vi "Disable_Enable.vi"(7 "Disabled":T2(ring)=enum."Disabled and Grayed Out", 8 "error in (no error)":errorcluster, 10 "Command":T1=enum."INIT", 11 "EpiWrapper in":refnum<class "EpiWrapper.lvclass">) -> (0 "error out":errorcluster, 3 "EpiWrapper out":refnum<class "EpiWrapper.lvclass">)   [LabVIEW 2012, in "EpiWrapper.lvclass"]
uses:
  EpiWrapper.lvclass
  Controls/Command_Enum.ctl
  Controls/Control_Selector.ctl
  Controls/Input_Selector.ctl
  EpiWrapper.lvclass/EpiWrapper.ctl
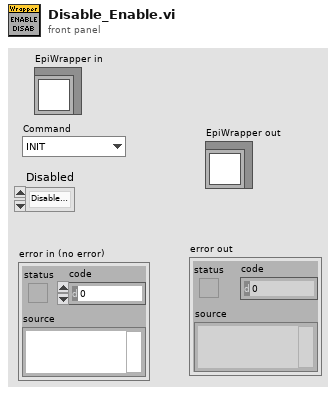
[diagram p1: front panel]
types:
  T1 = typedef "Command_Enum.ctl" = enum16{"RESETCONFIG", "OPENCONFIG", "RESET", "INIT", "LOAD", "MEASURE", "NEW", "SAVE", "UPDATE_INT", "SWAP_MODE", "UPDATE_ACQ", "EXIT", "CANCEL"}
  T2 = enum8{"Enabled", "Disabled", "Disabled and Grayed Out"}
  T3 = typedef "Input_Selector.ctl" = enum16{"Wafer ID", "Test", "New", "Save", "Load", "Cancel"}
  T4 = typedef "Control_Selector.ctl" = enum16{"Pass", "Fail", "Measure", "Area", "TestData"}
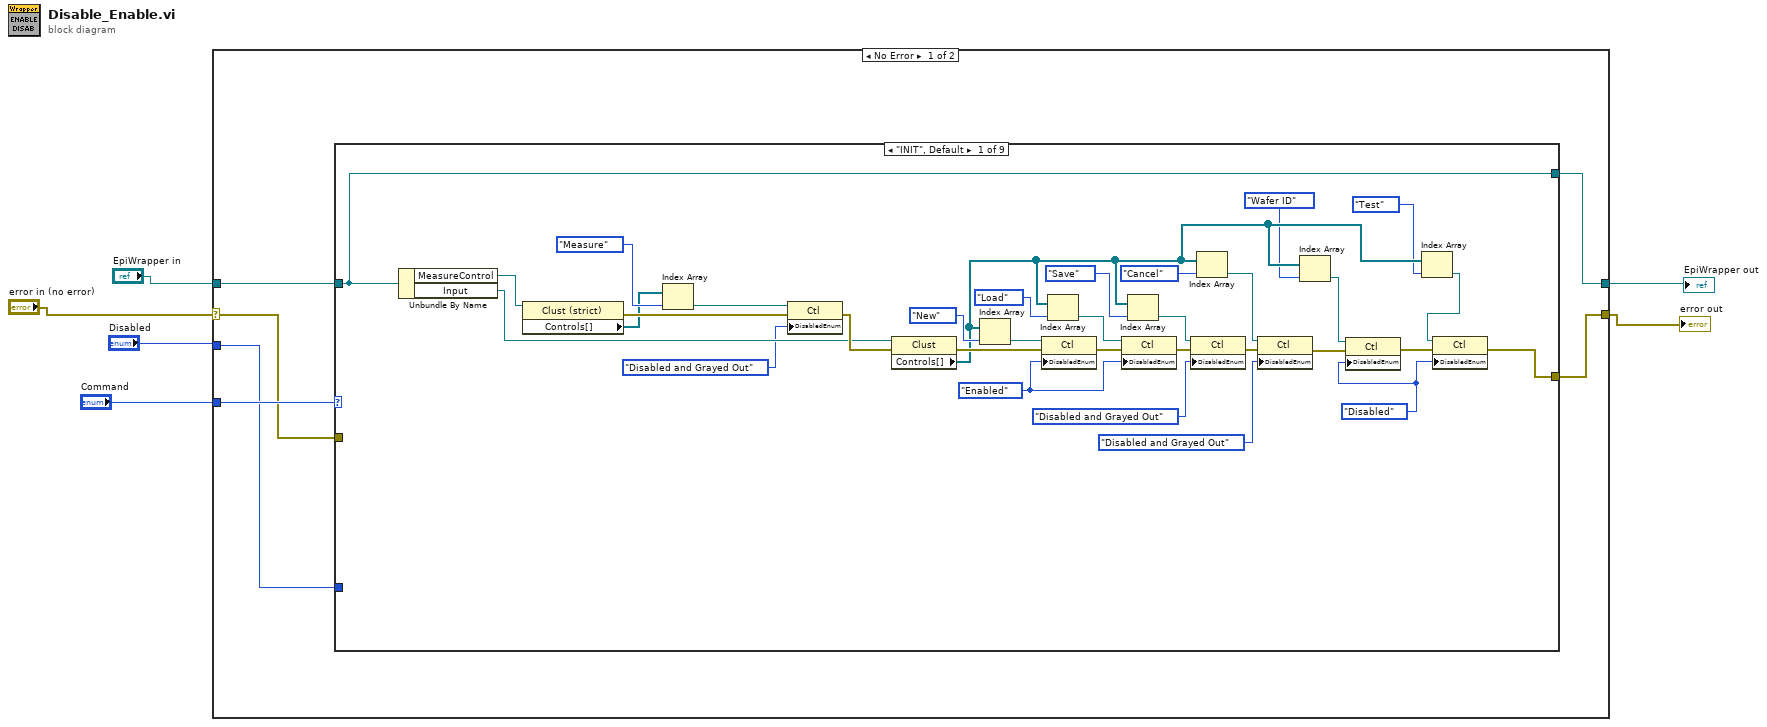
[diagram p0: block diagram]
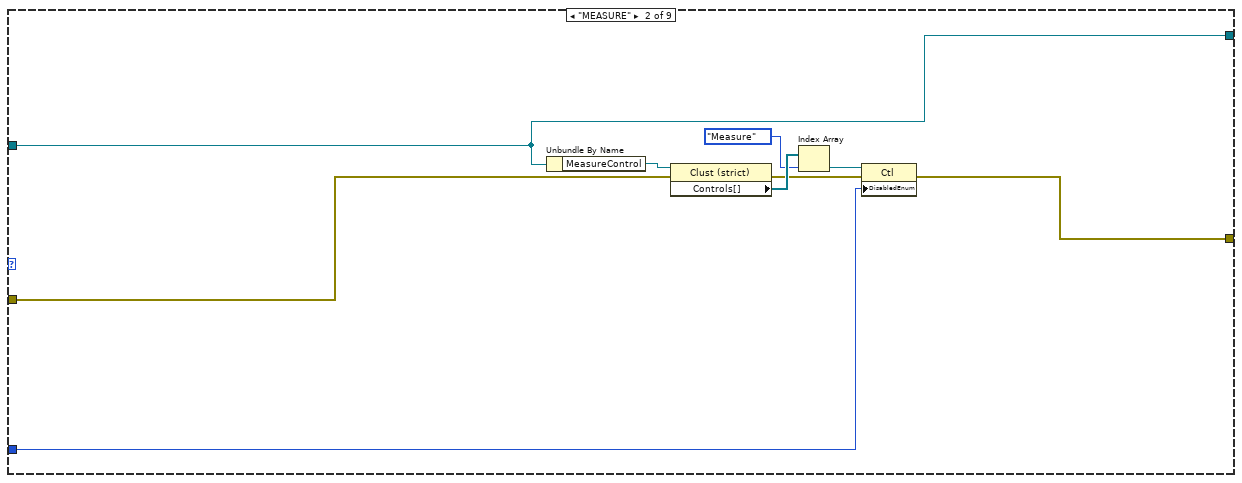
[diagram p2: hidden frame]
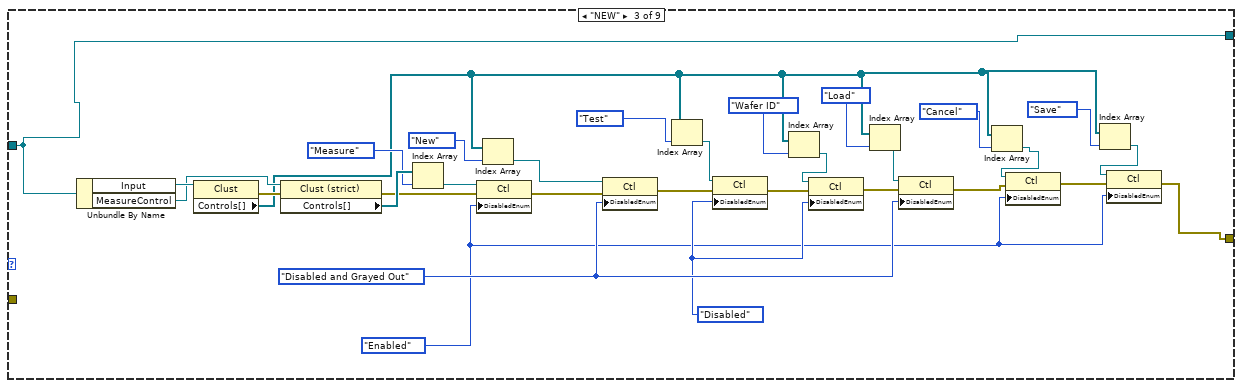
[diagram p3: hidden frame]
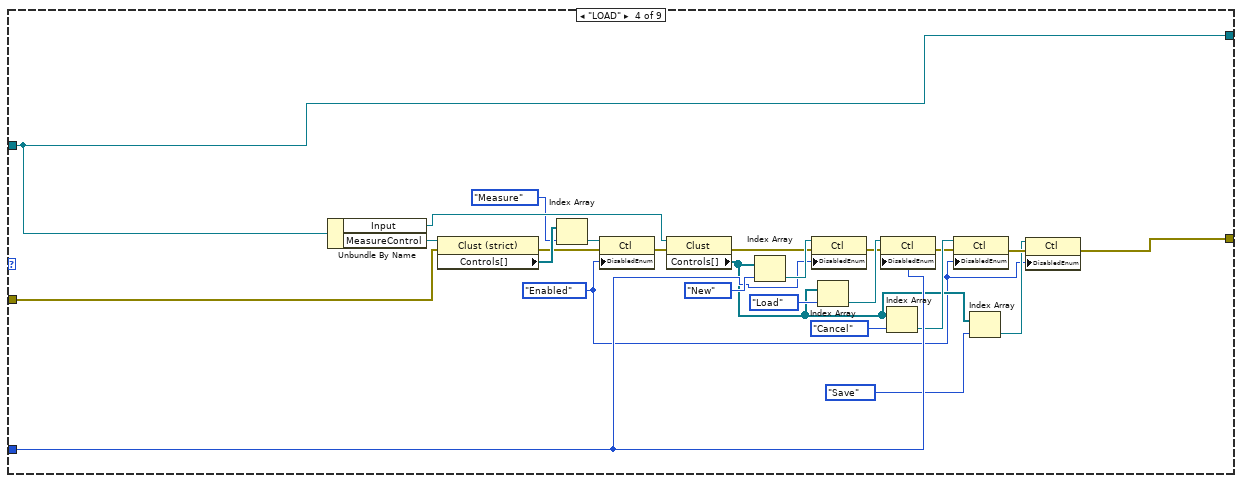
[diagram p4: hidden frame]
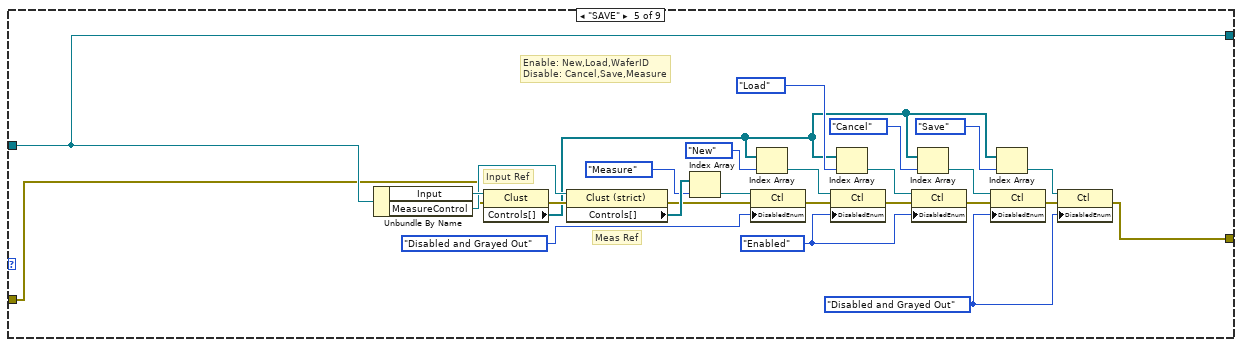
[diagram p5: hidden frame]
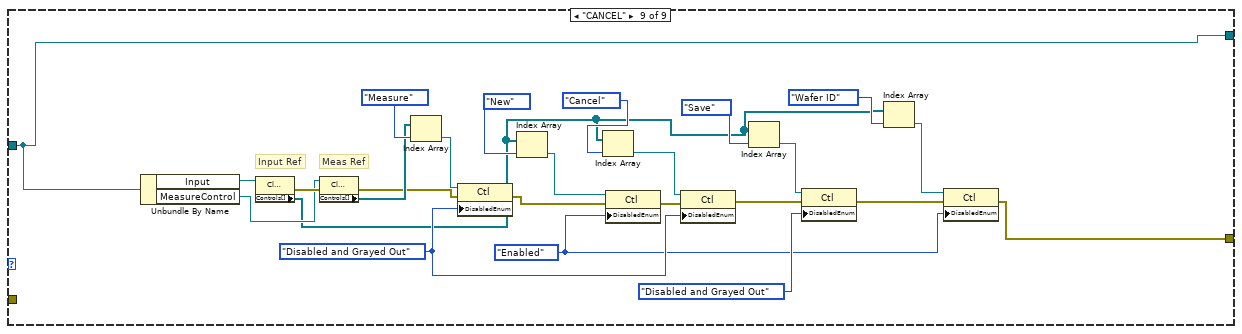
[diagram p9: hidden frame]
diagram:
  n1 = case shown="No Error" "error in (no error)" {
    selector: "error in (no error)" -> [w8 w169]
    tunnel: [w9 w169] -> w5
    tunnel: [w7 w168] -> w3
    tunnel: "EpiWrapper in" -> [w11 w168]
    tunnel: "Command" -> [w12 _]
    tunnel: "Disabled" -> [w10 _]
    frame No Error {
      n2 = case shown="\"INIT\", Default" w12 {
        tunnel: w11 -> [w35 w46 w72 w102 w118 w138 w140 w142 w155]
        tunnel: w10 -> [_ w47 _ w105 _ _ _ _ _]
        tunnel: [w18 w48 w55 w86 w111 w137 w139 w141 w143] -> w9
        tunnel: w8 -> [_ w50 _ w100 w117 w137 w139 w141 _]
        tunnel: [w35 w46 w72 w102 w118 w138 w140 w142 w155] -> w7
        frame "INIT", Default {
          w13 = T2."Disabled" ("Disabled")
          w24 = T2."Enabled" ("Disabled")
          n3 = Unbundle By Name(w35) -> ("MeasureControl"=w39:refnum<vi>, "Input"=w38:refnum<vi>)
          n4 = property class="Clust (strict)"(reference=w39) -> (error out=w42:errorcluster, "Controls[]"=w37:refnum<vi>[])  [unwired: 1 in, 1 out]
          n5 = Index Array(array=w37, index=Control_Selector."Measure" ("Control_Selector")) -> (element=w41:refnum<vi>)
          n6 = property class="Ctl"(reference=w41, error in=w42, "DisabledEnum"=T2."Disabled and Grayed Out" ("Disabled")) -> (error out=w45:errorcluster)  [unwired: 1 out]
          n7 = property class="Clust"(reference=w38, error in=w45) -> (error out=w28:errorcluster, "Controls[]"=w21:refnum<vi>[])  [unwired: 1 out]
          n8 = Index Array(array=w21, index=Input_Selector."New" ("InputSelector")) -> (element=w43:refnum<vi>)
          n9 = property class="Ctl"(reference=w43, error in=w28, "DisabledEnum"=w24) -> (error out=w23:errorcluster)  [unwired: 1 out]
          n10 = Index Array(array=w21, index=Input_Selector."Load" ("InputSelector")) -> (element=w25:refnum<vi>)
          n11 = property class="Ctl"(reference=w25, error in=w23, "DisabledEnum"=w24) -> (error out=w22:errorcluster)  [unwired: 1 out]
          n12 = Index Array(array=w21, index=Input_Selector."Save" ("InputSelector")) -> (element=w30:refnum<vi>)
          n13 = property class="Ctl"(reference=w30, error in=w22, "DisabledEnum"=T2."Disabled and Grayed Out" ("Disabled")) -> (error out=w27:errorcluster)  [unwired: 1 out]
          n14 = Index Array(array=w21, index=Input_Selector."Cancel" ("InputSelector")) -> (element=w29:refnum<vi>)
          n15 = property class="Ctl"(reference=w29, error in=w27, "DisabledEnum"=T2."Disabled and Grayed Out" ("Disabled")) -> (error out=w16:errorcluster)  [unwired: 1 out]
          n16 = Index Array(array=w21, index=Input_Selector."Wafer ID" ("InputSelector")) -> (element=w15:refnum<vi>)
          n17 = property class="Ctl"(reference=w15, error in=w16, "DisabledEnum"=w13) -> (error out=w17:errorcluster)  [unwired: 1 out]
          n18 = Index Array(array=w21, index=Input_Selector."Test" ("InputSelector")) -> (element=w14:refnum<vi>)
          n19 = property class="Ctl"(reference=w14, error in=w17, "DisabledEnum"=w13) -> (error out=w18:errorcluster)  [unwired: 1 out]
        }
        frame "MEASURE" {
          n20 = Unbundle By Name(w46) -> ("MeasureControl"=w53:refnum<vi>)
          n21 = property class="Clust (strict)"(reference=w53, error in=w50) -> (error out=w49:errorcluster, "Controls[]"=w54:refnum<vi>[])  [unwired: 1 out]
          n22 = Index Array(array=w54, index=Control_Selector."Measure" ("Control_Selector")) -> (element=w51:refnum<vi>)
          n23 = property class="Ctl"(reference=w51, error in=w49, "DisabledEnum"=w47) -> (error out=w48:errorcluster)  [unwired: 1 out]
        }
        frame "NEW" {
          w61 = T2."Disabled" ("Disabled")
          w64 = T2."Disabled and Grayed Out" ("Disabled")
          w57 = T2."Enabled" ("Disabled")
          n24 = Unbundle By Name(w72) -> ("Input"=w84:refnum<vi>, "MeasureControl"=w82:refnum<vi>)
          n25 = property class="Clust"(reference=w84) -> (error out=w81:errorcluster, "Controls[]"=w59:refnum<vi>[])  [unwired: 1 in, 1 out]
          n26 = property class="Clust (strict)"(reference=w82, error in=w81) -> (error out=w77:errorcluster, "Controls[]"=w80:refnum<vi>[])  [unwired: 1 out]
          n27 = Index Array(array=w80, index=Control_Selector."Measure" ("Control_Selector")) -> (element=w78:refnum<vi>)
          n28 = property class="Ctl"(reference=w78, error in=w77, "DisabledEnum"=w57) -> (error out=w76:errorcluster)  [unwired: 1 out]
          n29 = Index Array(array=w59, index=Input_Selector."New" ("InputSelector")) -> (element=w85:refnum<vi>)
          n30 = property class="Ctl"(reference=w85, error in=w76, "DisabledEnum"=w64) -> (error out=w69:errorcluster)  [unwired: 1 out]
          n31 = Index Array(array=w59, index=Input_Selector."Test" ("InputSelector")) -> (element=w70:refnum<vi>)
          n32 = property class="Ctl"(reference=w70, error in=w69, "DisabledEnum"=w61) -> (error out=w68:errorcluster)  [unwired: 1 out]
          n33 = Index Array(array=w59, index=Input_Selector."Wafer ID" ("InputSelector")) -> (element=w74:refnum<vi>)
          n34 = property class="Ctl"(reference=w74, error in=w68, "DisabledEnum"=w61) -> (error out=w65:errorcluster)  [unwired: 1 out]
          n35 = Index Array(array=w59, index=Input_Selector."Load" ("InputSelector")) -> (element=w66:refnum<vi>)
          n36 = property class="Ctl"(reference=w66, error in=w65, "DisabledEnum"=w64) -> (error out=w62:errorcluster)  [unwired: 1 out]
          n37 = Index Array(array=w59, index=Input_Selector."Cancel" ("InputSelector")) -> (element=w63:refnum<vi>)
          n38 = property class="Ctl"(reference=w63, error in=w62, "DisabledEnum"=w57) -> (error out=w56:errorcluster)  [unwired: 1 out]
          n39 = Index Array(array=w59, index=Input_Selector."Save" ("InputSelector")) -> (element=w60:refnum<vi>)
          n40 = property class="Ctl"(reference=w60, error in=w56, "DisabledEnum"=w57) -> (error out=w55:errorcluster)  [unwired: 1 out]
        }
        frame "LOAD" {
          w87 = T2."Enabled" ("Disabled")
          n41 = Unbundle By Name(w102) -> ("Input"=w109:refnum<vi>, "MeasureControl"=w101:refnum<vi>)
          n42 = property class="Clust (strict)"(reference=w101, error in=w100) -> (error out=w96:errorcluster, "Controls[]"=w99:refnum<vi>[])  [unwired: 1 out]
          n43 = Index Array(array=w99, index=Control_Selector."Measure" ("Control_Selector")) -> (element=w97:refnum<vi>)
          n44 = property class="Ctl"(reference=w97, error in=w96, "DisabledEnum"=w87) -> (error out=w95:errorcluster)  [unwired: 1 out]
          n45 = property class="Clust"(reference=w109, error in=w95) -> (error out=w103:errorcluster, "Controls[]"=w90:refnum<vi>[])  [unwired: 1 out]
          n46 = Index Array(array=w90, index=Input_Selector."New" ("InputSelector")) -> (element=w110:refnum<vi>)
          n47 = property class="Ctl"(reference=w110, error in=w103, "DisabledEnum"=w105) -> (error out=w104:errorcluster)  [unwired: 1 out]
          n48 = Index Array(array=w90, index=Input_Selector."Load" ("InputSelector")) -> (element=w106:refnum<vi>)
          n49 = property class="Ctl"(reference=w106, error in=w104, "DisabledEnum"=w105) -> (error out=w92:errorcluster)  [unwired: 1 out]
          n50 = Index Array(array=w90, index=Input_Selector."Cancel" ("InputSelector")) -> (element=w93:refnum<vi>)
          n51 = property class="Ctl"(reference=w93, error in=w92, "DisabledEnum"=w87) -> (error out=w91:errorcluster)  [unwired: 1 out]
          n52 = Index Array(array=w90, index=Input_Selector."Save" ("InputSelector")) -> (element=w88:refnum<vi>)
          n53 = property class="Ctl"(reference=w88, error in=w91, "DisabledEnum"=w87) -> (error out=w86:errorcluster)  [unwired: 1 out]
        }
        frame "SAVE" {
          w120 = T2."Enabled" ("Disabled")
          w112 = T2."Disabled and Grayed Out" ("Disabled")
          # "Enable: New,Load,WaferID\nDisable: Cancel,Save,Measure"
          # "Input Ref"
          # "Meas Ref"
          n54 = Unbundle By Name(w118) -> ("Input"=w135:refnum<vi>, "MeasureControl"=w133:refnum<vi>)
          n55 = property class="Clust"(reference=w135, error in=w117) -> (error out=w132:errorcluster, "Controls[]"=w116:refnum<vi>[])  [unwired: 1 out]
          n56 = property class="Clust (strict)"(reference=w133, error in=w132) -> (error out=w128:errorcluster, "Controls[]"=w131:refnum<vi>[])  [unwired: 1 out]
          n57 = Index Array(array=w131, index=Control_Selector."Measure" ("Control_Selector")) -> (element=w129:refnum<vi>)
          n58 = property class="Ctl"(reference=w129, error in=w128, "DisabledEnum"=T2."Disabled and Grayed Out" ("Disabled")) -> (error out=w127:errorcluster)  [unwired: 1 out]
          n59 = Index Array(array=w116, index=Input_Selector."New" ("InputSelector")) -> (element=w136:refnum<vi>)
          n60 = property class="Ctl"(reference=w136, error in=w127, "DisabledEnum"=w120) -> (error out=w119:errorcluster)  [unwired: 1 out]
          n61 = Index Array(array=w116, index=Input_Selector."Load" ("InputSelector")) -> (element=w125:refnum<vi>)
          n62 = property class="Ctl"(reference=w125, error in=w119, "DisabledEnum"=w120) -> (error out=w122:errorcluster)  [unwired: 1 out]
          n63 = Index Array(array=w116, index=Input_Selector."Cancel" ("InputSelector")) -> (element=w123:refnum<vi>)
          n64 = property class="Ctl"(reference=w123, error in=w122, "DisabledEnum"=w112) -> (error out=w113:errorcluster)  [unwired: 1 out]
          n65 = Index Array(array=w116, index=Input_Selector."Save" ("InputSelector")) -> (element=w114:refnum<vi>)
          n66 = property class="Ctl"(reference=w114, error in=w113, "DisabledEnum"=w112) -> (error out=w111:errorcluster)  [unwired: 1 out]
        }
        frame "SWAP_MODE" {
        }
        frame "UPDATE_ACQ" {
        }
        frame "EXIT" {
        }
        frame "CANCEL" {
          w144 = T2."Enabled" ("Disabled")
          w151 = T2."Disabled and Grayed Out" ("Disabled")
          # "Meas Ref"
          # "Input Ref"
          n67 = Unbundle By Name(w155) -> ("Input"=w167:refnum<vi>, "MeasureControl"=w160:refnum<vi>)
          n68 = property class="Clust"(reference=w167) -> (error out=w161:errorcluster, "Controls[]"=w145:refnum<vi>[])  [unwired: 1 in, 1 out]
          n69 = property class="Clust (strict)"(reference=w160, error in=w161) -> (error out=w158:errorcluster, "Controls[]"=w159:refnum<vi>[])  [unwired: 1 out]
          n70 = Index Array(array=w159, index=Control_Selector."Measure" ("Control_Selector")) -> (element=w157:refnum<vi>)
          n71 = property class="Ctl"(reference=w157, error in=w158, "DisabledEnum"=w151) -> (error out=w156:errorcluster)  [unwired: 1 out]
          n72 = Index Array(array=w145, index=Input_Selector."New" ("InputSelector")) -> (element=w154:refnum<vi>)
          n73 = Index Array(array=w145, index=Input_Selector."Cancel" ("InputSelector")) -> (element=w152:refnum<vi>)
          n74 = property class="Ctl"(reference=w154, error in=w156, "DisabledEnum"=w144) -> (error out=w163:errorcluster)  [unwired: 1 out]
          n75 = property class="Ctl"(reference=w152, error in=w163, "DisabledEnum"=w151) -> (error out=w148:errorcluster)  [unwired: 1 out]
          n76 = Index Array(array=w145, index=Input_Selector."Save" ("InputSelector")) -> (element=w150:refnum<vi>)
          n77 = property class="Ctl"(reference=w150, error in=w148, "DisabledEnum"=T2."Disabled and Grayed Out" ("Disabled")) -> (error out=w147:errorcluster)  [unwired: 1 out]
          n78 = Index Array(array=w145, index=Input_Selector."Wafer ID" ("InputSelector")) -> (element=w146:refnum<vi>)
          n79 = property class="Ctl"(reference=w146, error in=w147, "DisabledEnum"=w144) -> (error out=w143:errorcluster)  [unwired: 1 out]
        }
      }
    }
    frame Error {
    }
  }
  "error out" <- w5
  "EpiWrapper out" <- w3
